vi "Ball Get Next State.vi"(11 "Ball Main Cluster in":T2={"Ball FIFO"=[], "Camera Name"="", "Ball path"=path "", "Control Ref's"=[], "Greyscale Mask Image"=refnum, "Main Image"=refnum, "Algae Color Range"={"Hue"={21.620689392089844, 69.62068939208984}, "Sat"={66.41378784179688, 255.0}, "Val"={96.0, 255.0}}, "Timeout"=5, "EDIT Settings"=FALSE}) -> (1 "Next State":T1, 3 "Ball Main Cluster out":T2={"Ball FIFO"=[], "Camera Name"="", "Ball path"=path "", "Control Ref's"=[], "Greyscale Mask Image"=refnum, "Main Image"=refnum, "Algae Color Range"={"Hue"={21.620689392089844, 69.62068939208984}, "Sat"={66.41378784179688, 255.0}, "Val"={96.0, 255.0}}, "Timeout"=5, "EDIT Settings"=FALSE})   [LabVIEW 2025]
uses:
  Ball Main CLuster.ctl
  Ball States.ctl
  <vilib>/vision/Image Controls.llb/IMAQ Image.ctl
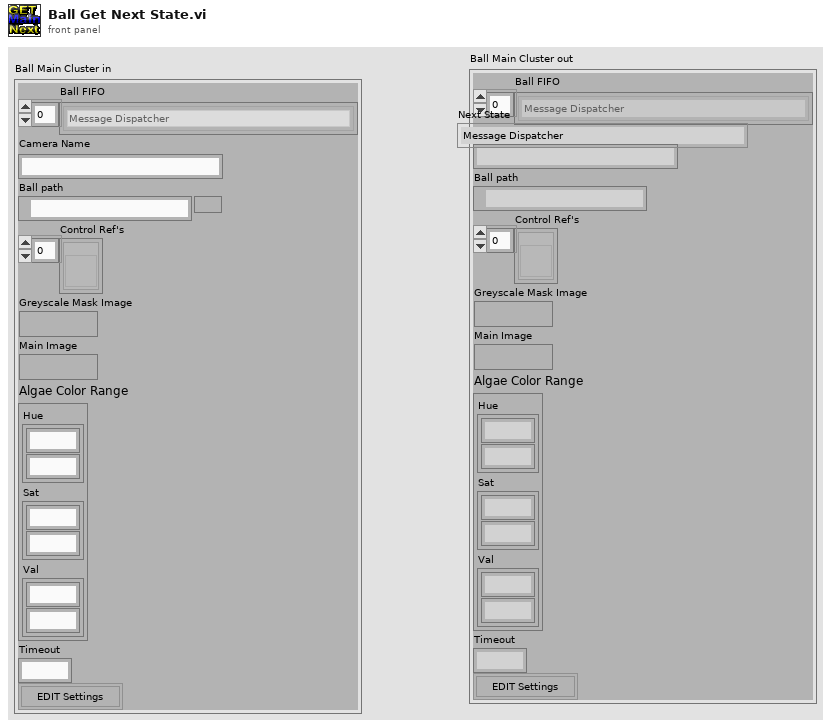
[diagram p1: front panel]
types:
  T1 = typedef "Ball States.ctl" = enum16{"Message Dispatcher", "INI", "Open", "Save", "Exit"}
  T2 = typedef "Ball Main CLuster.ctl" = cluster{"Ball FIFO":T1[], "Camera Name":string, "Ball path":path, "Control Ref's":refnum<vi>[], "Greyscale Mask Image":T3, "Main Image":T3, "Algae Color Range":cluster{"Hue":cluster{dbl, dbl}, "Sat":cluster{dbl, dbl}, "Val":cluster{dbl, dbl}}, "Timeout":i32, "EDIT Settings":bool}
  T3 = typedef "IMAQ Image.ctl" = refnum<image>
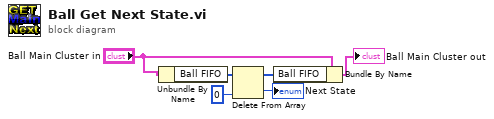
[diagram p0: block diagram]
diagram:
  n1 = Unbundle By Name("Ball Main Cluster in") -> ("Ball FIFO"=w6:T1[])
  n2 = Delete From Array(array=w6, index=0) -> (deleted portion=→"Next State":T1, array with subset deleted=w3:T1[])  [unwired: 1 in]
  n3 = Bundle By Name(cluster="Ball Main Cluster in", "Ball FIFO"=w3) -> (→"Ball Main Cluster out":T2)
